vi "shift register adding up.vi"() -> ()   [LabVIEW 2016]
panel:
  out "Sum":i32
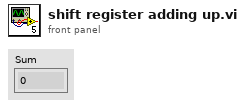
[diagram p1: front panel]
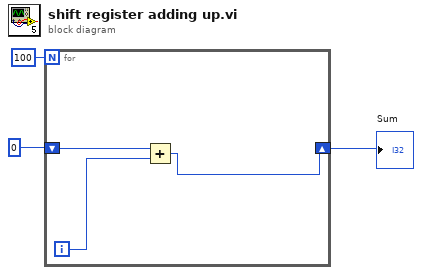
[diagram p0: block diagram]
diagram:
  n1 = for {
    N: 100 -> [_]
    shift-right: [w6] -> w1
    shift-left: 0 -> [w5]
    i -> [w4]
    n2 = Add(x=w5, y=w4) -> (x+y=w6:i32)
  }
  "Sum" <- w1
